vi "sub1.vi"() -> (2 "String":string)   [LabVIEW 2013]
panel:
  in  "stato 3":bool
  in  "stato 2":bool
  in  "stop":bool
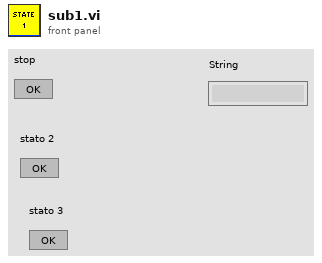
[diagram p1: front panel]
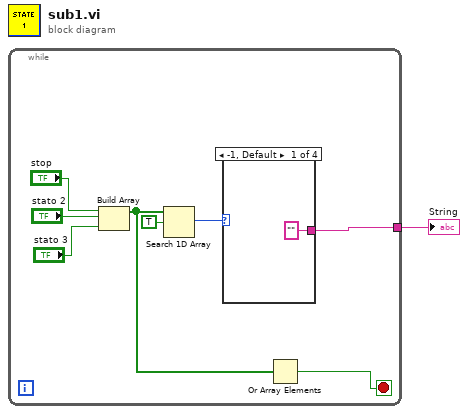
[diagram p0: block diagram]
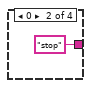
[diagram p2: hidden frame]
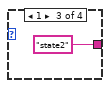
[diagram p3: hidden frame]
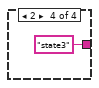
[diagram p4: hidden frame]
diagram:
  n1 = while {
    tunnel: [w9] -> w1
    stop <- w3 stop-if-true
    n2 = Build Array("stop", "stato 2", "stato 3") -> (w2:bool[])
    n3 = Search 1D Array(1D array=w2, element=TRUE) -> (index of element=w8:i32)  [unwired: 1 in]
    n4 = case shown="-1, Default" w8 {
      tunnel: ["" "stop" "state2" "state3"] -> w9
      frame -1, Default {
      }
      frame 0 {
      }
      frame 1 {
      }
      frame 2 {
      }
    }
    n5 = Or Array Elements(Boolean array=w2) -> (logical OR=w3:bool)
  }
  "String" <- w1
